vi "Write Marker Values[].vi"(5 "Marker Values[]":cluster{dbl, u32}[](array[cluster]), 9 "ColorScale in":refnum<class "ColorScale.lvclass">) -> (3 "ColorScale out":refnum<class "ColorScale.lvclass">)   [LabVIEW 2014, in "Raspberry Pi Compatible Compiler for LabVIEW.lvlib" / "ColorScale.lvclass"]
uses:
  ColorScale.lvclass
  ColorScale.lvclass/ColorScale.ctl
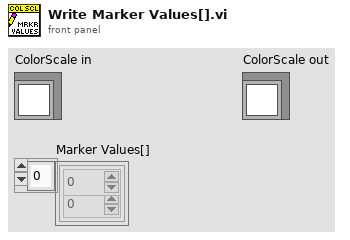
[diagram p1: front panel]
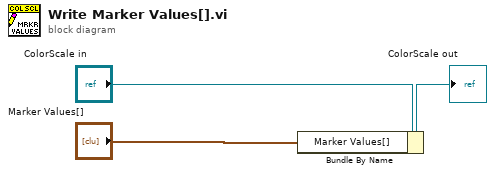
[diagram p0: block diagram]
diagram:
  n1 = Bundle By Name(cluster="ColorScale in", "Marker Values[]"="Marker Values[]") -> (→"ColorScale out":refnum<class "ColorScale.lvclass">)
